vi "GetTeamListFromFRC.vi"() -> ()   [LabVIEW 2018]
uses:
  <vilib>/Utility/config.llb/Write Key (String).vi
  <vilib>/Utility/config.llb/NI_LVConfig.lvlib
panel:
  in  "Update Scouting File":bool
  out "Select":string
  out "Teams":T1(array[cluster])
  in  "Event":string(combo)
  out "innerText":string
  in  "WebBrowser":refnum<k7>(container)
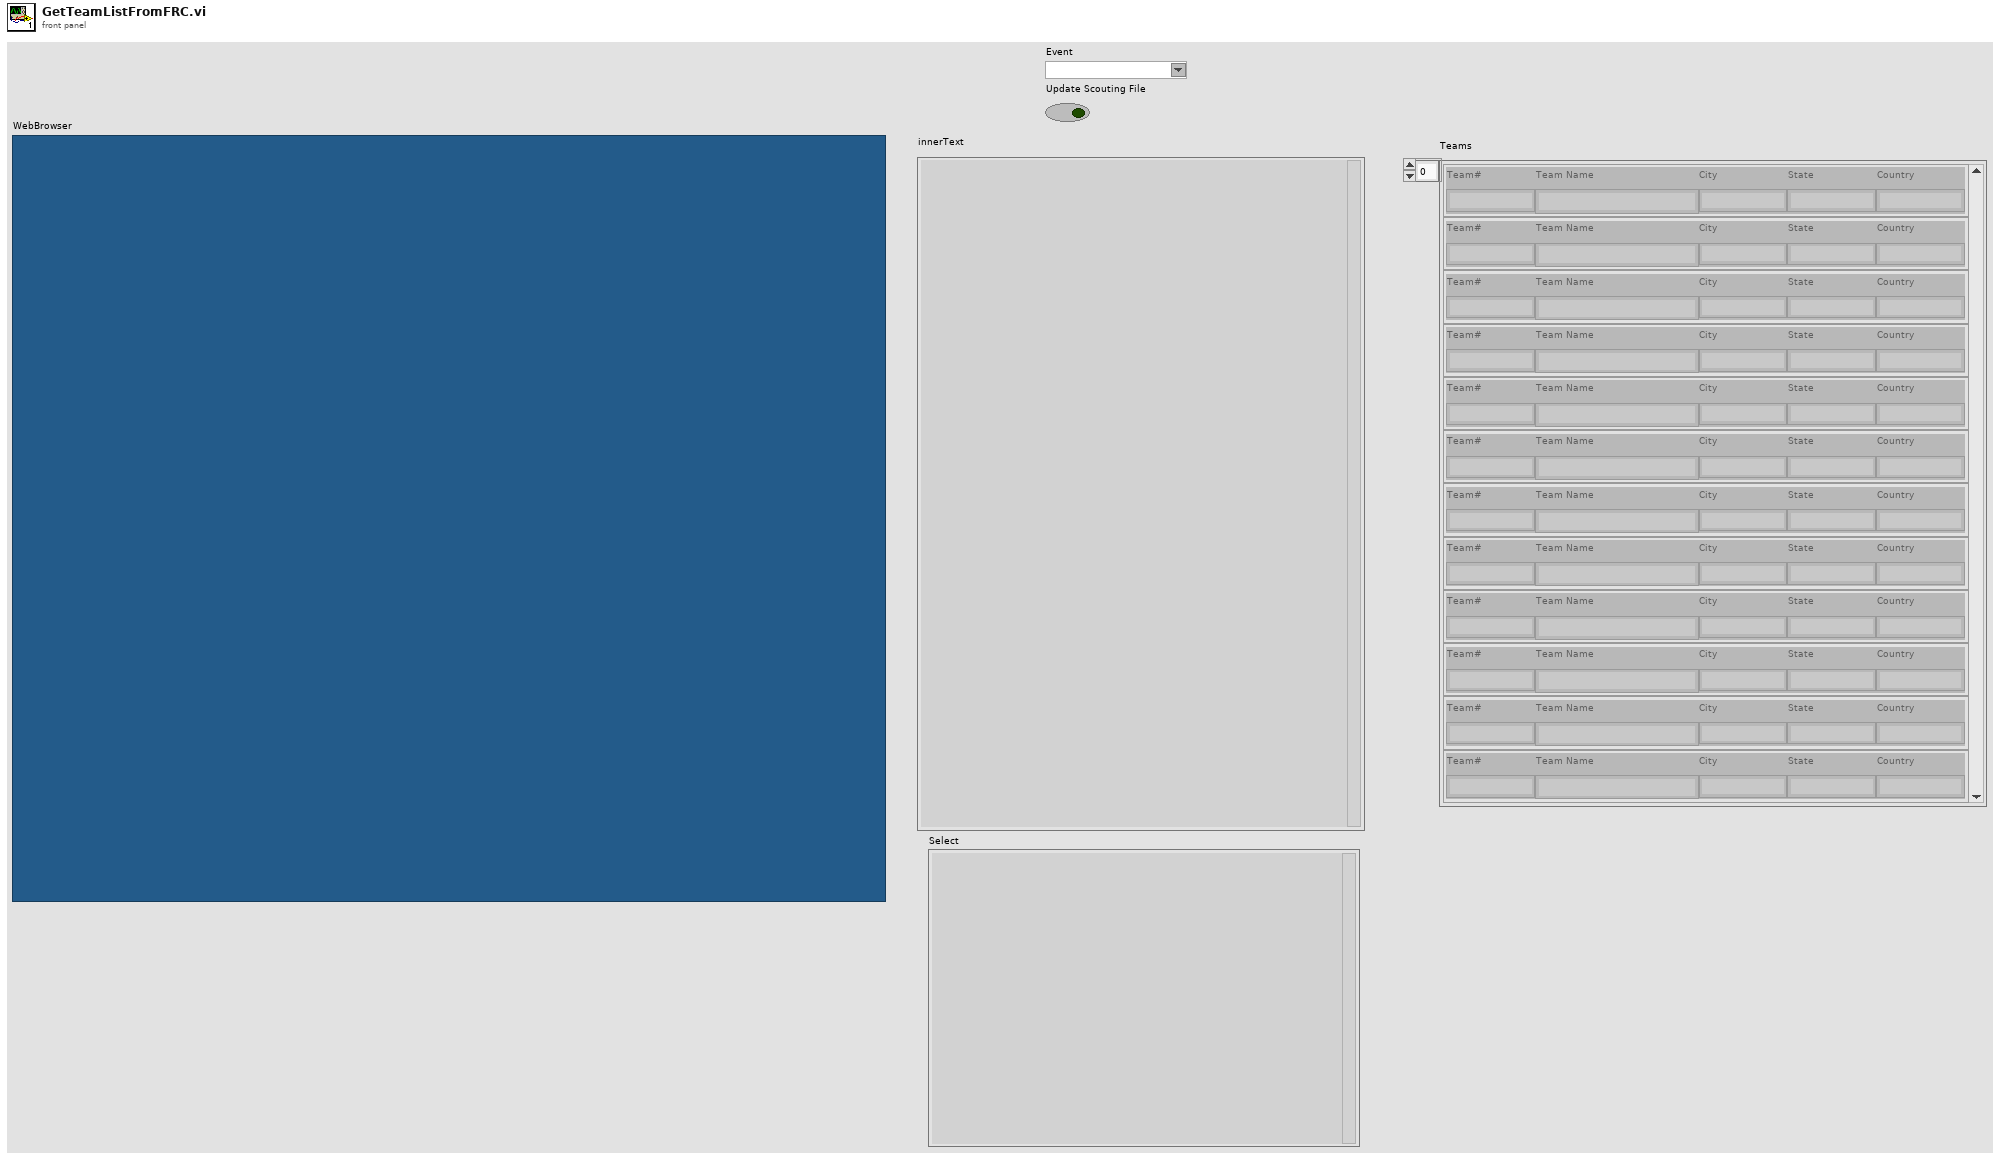
[diagram p1: front panel]
types:
  T1 = cluster{"Team#":string, "Team Name":string, "City":string, "State":string, "Country":string}[]
  T2 = cluster{"Team#":string, "Team Name":string, "City":string, "State":string, "Country":string}
  T3 = typedef "NI_LVConfig.lvlib/Config Data RefNum.ctl" = refnum<k1>
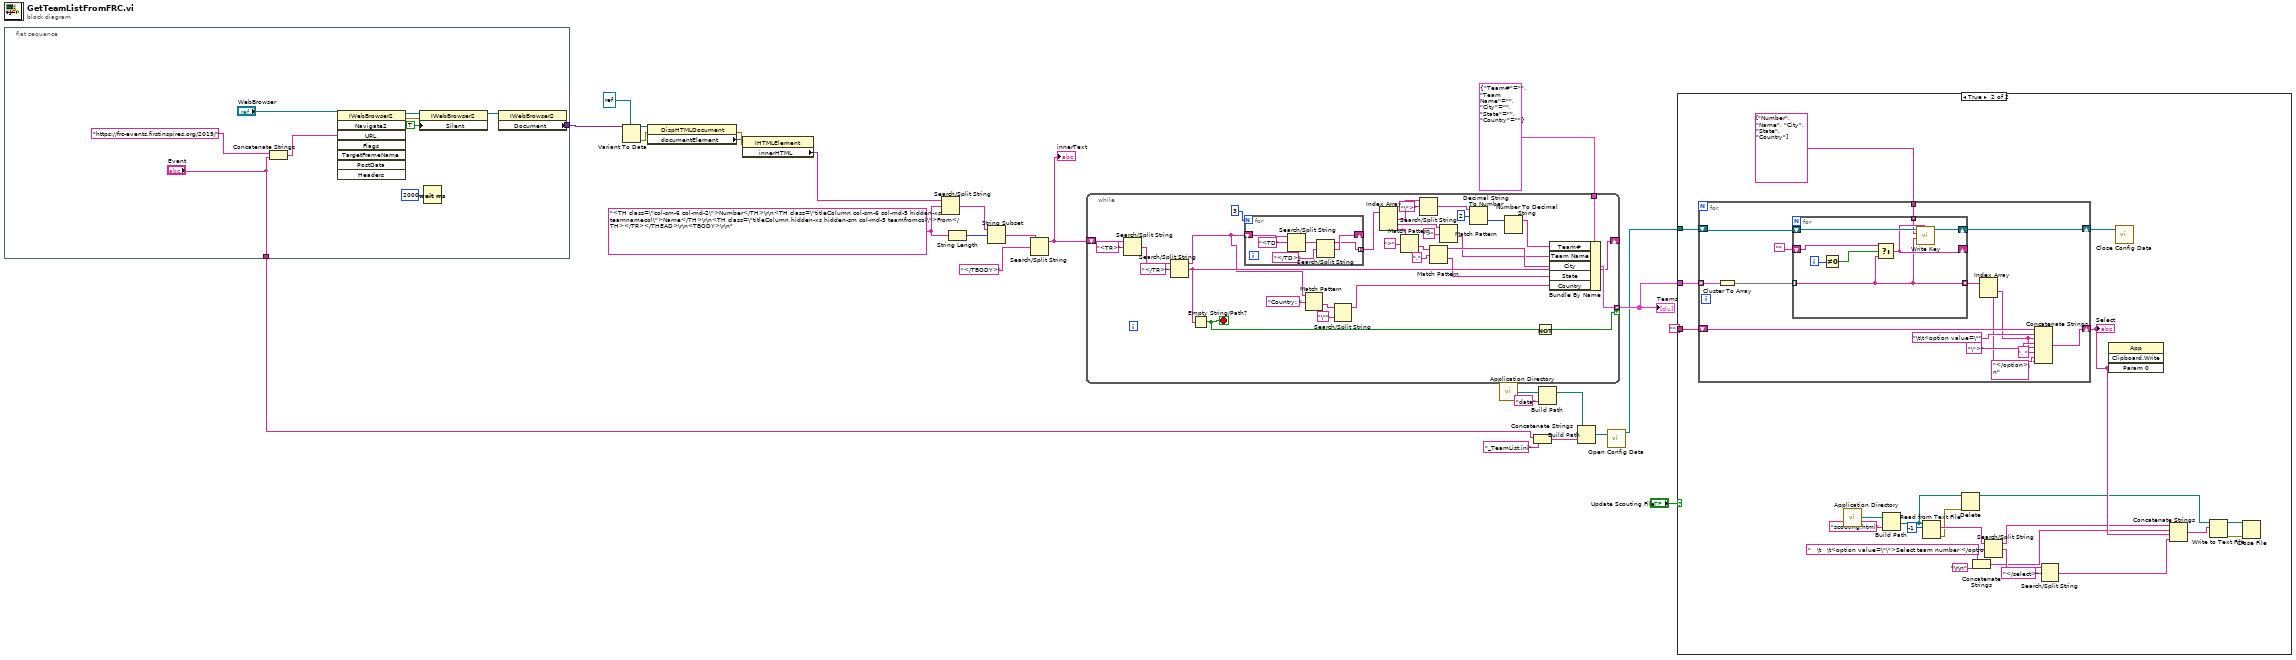
[diagram p0: block diagram]
diagram:
  w15 = "<TH class=\"col-sm-6 col-md-2\">Number</TH>\r\n<TH class=\"titleColumn col-sm-6 col-md-5 hidden-xs teamnamecol\">Name</TH>\r\n<TH class=\"titleColumn hidden-xs hidden-sm col-md-5 teamfromcol\">From</TH></TR></THEAD>\r\n<TBODY>\r\n" ("search string/char (-)")
  n1 = flat-sequence {
    tunnel: [w35] -> w25
    tunnel: ["Event"] -> w8
    frame #0 {
      n2 = Concatenate Strings("https://frc-events.firstinspires.org/2019/", "Event") -> (w29:string)
      n3 = invoke class="IWebBrowser2" method="Navigate2"(reference="WebBrowser", "URL"=w29) -> (reference out=w31:refnum<k7>, error out=w33:errorcluster)  [unwired: 6 in, 6 out]
      n4 = property class="IWebBrowser2"(reference=w31, error in=w33, "Silent"=TRUE) -> (reference out=w34:refnum<k7>)  [unwired: 1 out]
      n5 = Wait (ms)(milliseconds to wait=u32 2000) -> ()  [unwired: 1 out]
      n6 = property class="IWebBrowser2"(reference=w34) -> ("Document"=w35:variant)  [unwired: 1 in, 2 out]
    }
  }
  n7 = Variant To Data(type=refnum<k7> refnum ("reference out"), Variant=w25) -> (data=w20:refnum<k7>, error out=w23:errorcluster)  [unwired: 1 in]
  n8 = property class="DispHTMLDocument"(reference=w20, error in=w23) -> (error out=w24:errorcluster, "documentElement"=w22:refnum<k7>)  [unwired: 1 out]
  n9 = property class="IHTMLElement"(reference=w22, error in=w24) -> ("innerHTML"=w19:string)  [unwired: 2 out]
  n10 = Search/Split String(string=w19, search string/char (-)=w15) -> (match + rest of string=w16:string)  [unwired: 1 in, 2 out]
  n11 = String Length(string=w15) -> (length=w14:i32)
  n12 = String Subset(string=w16, offset (0)=w14) -> (substring=w13:string)  [unwired: 1 in]
  n13 = Search/Split String(string=w13, search string/char (-)="</TBODY>") -> (substring before match=w17:string)  [unwired: 1 in, 2 out]
  "innerText" <- w17
  n14 = while {
    shift-right: [w60] -> _
    shift-left: w17 -> [w66]
    tunnel: T2 {"Team#"="", "Team Name"="", "City"="", "State"="", "Country"=""} -> [w62]
    tunnel: [w61] -> w10 mode=indexing if=w59
    stop <- w39 stop-if-true
    n15 = Search/Split String(string=w66, search string/char (-)="<TR>") -> (match + rest of string=w64:string)  [unwired: 1 in, 2 out]
    n16 = Search/Split String(string=w64, search string/char (-)="</TR>") -> (substring before match=w42:string, match + rest of string=w60:string)  [unwired: 1 in, 1 out]
    n17 = Empty String/Path?(string/path=w60) -> (empty?=w39:bool)
    n18 = for {
      N: 3 -> [_]
      shift-right: [w68] -> _
      shift-left: w42 -> [w72]
      tunnel: [w67] -> w55 mode=indexing
      n19 = Search/Split String(string=w72, search string/char (-)="<TD") -> (match + rest of string=w70:string)  [unwired: 1 in, 2 out]
      n20 = Search/Split String(string=w70, search string/char (-)="</TD>") -> (substring before match=w67:string, match + rest of string=w68:string)  [unwired: 1 in, 1 out]
    }
    n21 = Match Pattern(string=w42, regular expression="Country: ") -> (after substring=w41:string)  [unwired: 1 in, 3 out]
    n22 = Search/Split String(string=w41, search string/char (-)="\"") -> (substring before match=w36:string)  [unwired: 1 in, 2 out]
    n23 = Index Array(array=w55) -> (element #1=w53:string, element #2=w47:string, element #3=w45:string)  [unwired: 3 in]
    n24 = Match Pattern(string=w45, regular expression=">") -> (after substring=w44:string)  [unwired: 1 in, 3 out]
    n25 = Search/Split String(string=w53, search string/char (-)="\">") -> (match + rest of string=w52:string)  [unwired: 1 in, 2 out]
    n26 = Match Pattern(string=w44, regular expression=",") -> (before substring=w50:string, after substring=w37:string)  [unwired: 1 in, 2 out]
    n27 = Match Pattern(string=w47, regular expression=">") -> (after substring=w49:string)  [unwired: 1 in, 3 out]
    n28 = Decimal String To Number(string=w52, offset=2) -> (number=w57:i32)  [unwired: 1 in, 1 out]
    n29 = Number To Decimal String(number=w57) -> (decimal integer string=w38:string)  [unwired: 1 in]
    n30 = Not(x=w39) -> (.not. x?=w59:bool)
    n31 = Bundle By Name(cluster=w62, "Team#"=w38, "Team Name"=w49, "City"=w50, "State"=w37, "Country"=w36) -> (w61:T2)
  }
  "Teams" <- w10
  n32 = call <vilib>:"Application Directory.vi"() -> ("Application Directory"=w4:path)
  n33 = Concatenate Strings(w8, "_TeamList.ini" ("string")) -> (w6:string)
  n34 = Build Path(base path=w4, name or relative path="data") -> (appended path=w3:path)
  n35 = Build Path(base path=w3, name or relative path=w6) -> (appended path=w7:path)
  n36 = call <vilib>:"Open Config Data.vi"("configuration file path"=w7) -> ("refnum"=w5:T3)  [unwired: 8 in, 2 out]
  n37 = case shown="True" "Update Scouting File" {
    tunnel: "" -> [_ w93]
    tunnel: w10 -> [_ w92]
    tunnel: w5 -> [_ w91]
    frame False {
    }
    frame True {
      w82 = "   \t   \t<option value=\"\">Select team number </option>" ("search string/char (-)")
      n38 = for {
        tunnel: w92 -> [w97] mode=indexing
        shift-right: [w108] -> w95
        shift-left: w91 -> [w110]
        tunnel: string[] ["Number", "Name", "City", "State", "Country"] -> [w107]
        shift-right: [w105] -> w84
        shift-left: w93 -> [w106]
        n39 = Cluster To Array(cluster=w97) -> (array=w96:string[])
        n40 = for {
          tunnel: w96 -> [w111] mode=indexing
          shift-right: [w114] -> _
          shift-left: "" -> [w115]
          shift-right: [w113] -> w108
          shift-left: w110 -> [w118]
          tunnel: w107 -> [w112] mode=indexing
          tunnel: [w111] -> w103 mode=indexing
          i -> [w117]
          n41 = Not Equal To 0?(x=w117) -> (x != 0?=w116:bool)
          n42 = Select(t=w115, s=w116, f=w111) -> (s? t:f=w114:string)
          n43 = call-poly <vilib>:"Write Key.vi"("section"=w114, "value"=w111, "key"=w112, "refnum"=w118) -> ("refnum out"=w113:T3)  [unwired: 5 in, 2 out]
        }
        n44 = Index Array(array=w103) -> (element #1=w101:string, element #2=w99:string)  [unwired: 2 in]
        n45 = Concatenate Strings(w106, "\t\t<option value=\"", w101, "\">" ("string"), w101, ", " ("string"), w99, "</option>\n" ("string")) -> (w105:string)
      }
      "Select" <- w84
      n46 = call <vilib>:"Application Directory.vi"() -> ("Application Directory"=w89:path)
      n47 = Build Path(base path=w89, name or relative path="scouting.html") -> (appended path=w73:path)
      n48 = Read from Text File(file (use dialog)=w73, count=-1) -> (text=w87:string, error out=w74:errorcluster)  [unwired: 2 in, 2 out]
      n49 = Delete(path (use dialog)=w73, error in=w74) -> (deleted path=w75:path)  [unwired: 3 in, 2 out]
      n50 = Concatenate Strings(w82, "\r\n") -> (w80:string)
      n51 = Search/Split String(string=w87, search string/char (-)=w82) -> (substring before match=w83:string, match + rest of string=w86:string)  [unwired: 1 in, 1 out]
      n52 = Search/Split String(string=w86, search string/char (-)="</select>") -> (match + rest of string=w81:string)  [unwired: 1 in, 2 out]
      n53 = invoke class="App" method="Clipboard.Write"("Param 0"=w84) -> ()  [unwired: 3 in, 4 out]
      n54 = call <vilib>:"Close Config Data.vi"("refnum"=w95) -> ()  [unwired: 9 in, 2 out]
      n55 = Concatenate Strings(w83, w80, w84, w81) -> (w78:string)
      n56 = Write to Text File(file (use dialog)=w75, text=w78) -> (refnum out=w76:refnum<file>, error out=w77:errorcluster)  [unwired: 2 in, 1 out]
      n57 = Close File(refnum=w76, error in=w77) -> ()  [unwired: 2 out]
    }
  }
